vi "Introspection Core.vi"(8 "error in (no error)":errorcluster, 11 "CS++ObjectManager in":refnum<class "CS++ObjectManager.lvclass">) -> (0 "error out":errorcluster, 2 "CS++Messages":refnum<class "Message.lvclass">[](array[class]), 3 "CS++ObjectManager out":refnum<class "CS++ObjectManager.lvclass">)   [LabVIEW 2014, in "CS++ObjectManager.lvlib" / "CS++ObjectManager.lvclass"]
doc: "This vi delivers a list with all messages this actor reacts to. \n\nNote that all inherited classes have to overwrite it."
uses:
  CS++ObjectManager.lvclass
  <vilib>/ActorFramework/Message/Message.lvclass
  CS++ObjectManager Messages/Update Actor List Msg/Update Actor List Msg.lvclass
  CSPP_Core/Actors/CS++GUIActor/CS++GUIActor.lvclass
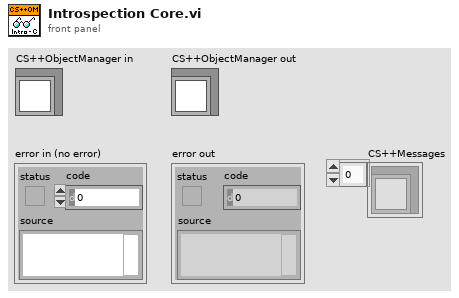
[diagram p1: front panel]
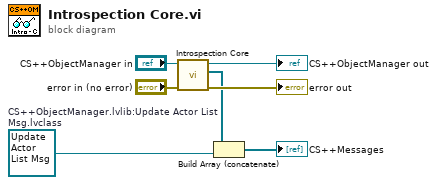
[diagram p0: block diagram]
diagram:
  w1 = refnum<class "Update Actor List Msg.lvclass"> refnum  # CS++ObjectManager.lvlib:Update Actor List Msg.lvclass
  n1 = call-parent "Introspection Core.vi"("error in (no error)"="error in (no error)", "CS++BaseActor in"="CS++ObjectManager in") -> ("error out"=→"error out":errorcluster, "CS++Messages"=w6:refnum<class "Message.lvclass">[], "CS++BaseActor out"=→"CS++ObjectManager out":refnum<class "CS++ObjectManager.lvclass">)  [unwired: 7 in]
  n2 = Build Array (concatenate)(w6, w1) -> (→"CS++Messages":refnum<class "Message.lvclass">[])
